vi "Robot Global Data.vi"() -> ()   [LabVIEW 2018]
doc: "This global VI can contain as many global variables as you need. Place a control on the panel, give it a good name. To read or write to it from a VI, drag the icon to the diagram of that VI. You can also drag from the project. Click on the node to change which global you access. You shouldn't have multiple locations writing to a global or it will cause a race-condition."
uses:
  <vilib>/Rock Robotics/WPI/Camera/WPI_CameraImageSize.ctl
  <vilib>/Rock Robotics/WPI/DriverStation/WPI_DriverStationRobotMode2.ctl
  Infrastructure/Joystick Controls.ctl
  Drivebase/Drive Motion Magic Setpoints.ctl
  <vilib>/Rock Robotics/WPI/ThirdParty/Phoenix-LabVIEW/Motor Controller/Controls/CTRE_Phoenix_MotorControl_ControlMode.ctl
panel:
  out "4bar setpoint/immediate value":T2 {"Control Mode" items=["PercentOutput"=0, "Position"=1, "Velocity"=2, "Current"=3, "Follower"=5, "MotionProfile"=6, "MotionMagic"=7, "MotionProfileArc"=10, "Disabled"=15]}
  in  "Drive Motor Values":T3
  in  "Manual Has Overridden Auton":bool
  in  "Drive MM Setpoints":T4
  in  "Step Auton Drive has Completed":i32
  in  "Joystick Controls":T5={"Driver Left Joystick X"=0.0, "Driver Left Joystick Y"=0.0, "Driver A Button"=FALSE, "Driver B Button"=FALSE, "Driver X Button"=FALSE, "Driver Y Button"=FALSE, "Driver Left Bumper"=FALSE, "Driver Right Bumper"=FALSE, "Driver View Button"=FALSE, "Driver Menu Button"=FALSE, "Driver Left Joystick Press"=FALSE, "Driver Right Joystick Press"=FALSE, "Driver Left Trigger"=0.0, "Driver Right Joystick X"=0.0, "Driver Right Joystick Y"=0.0, "Driver Right Trigger"=0.0, "Operator Left Joystick X"=0.0, "Operator Left Joystick Y"=0.0, "Operator A Button"=FALSE, "Operator B Button"=FALSE, "Operator X Button"=FALSE, "Operator Y Button"=FALSE, "Operator Left Bumper"=FALSE, "Operator Right Bumper"=FALSE, "Operator View Button"=FALSE, "Operator Menu Button"=FALSE, "Operator Left Joystick Press"=FALSE, "Operator Right Joystick Press"=FALSE, "Operator Left Trigger"=0.0, "Operator Right Joystick X"=0.0, "Operator Right Joystick Y"=0.0, "Operator Right Trigger"=0.0, "Driver D-Pad"=-1, "Operator D-Pad"=-1}
  in  "Robot Mode":T6
  in  "image size":T7=enum."320x240"
  in  "Enable Vision":bool
  # "AUTON"
  # "Typedef\nWriten to in Autonomous independant"
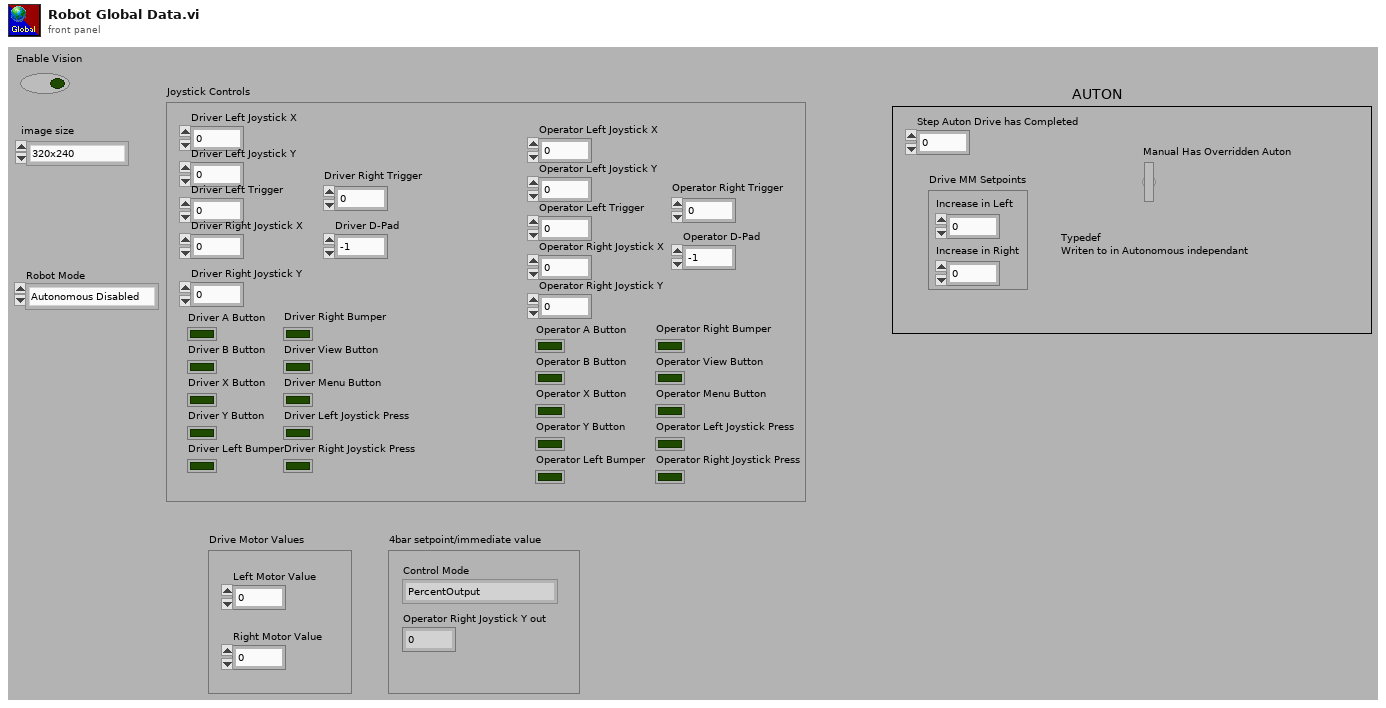
[diagram p1: front panel]
types:
  T1 = typedef "CTRE_Phoenix_MotorControl_ControlMode.ctl" = u16
  T2 = cluster{"Control Mode":T1, "Operator Right Joystick Y out":dbl}
  T3 = cluster{"Left Motor Value":dbl, "Right Motor Value":dbl}
  T4 = typedef "Drive Motion Magic Setpoints.ctl" = cluster{"Increase in Left":dbl, "Increase in Right":dbl}
  T5 = typedef "Joystick Controls.ctl" = cluster{"Driver Left Joystick X":dbl, "Driver Left Joystick Y":dbl, "Driver A Button":bool, "Driver B Button":bool, "Driver X Button":bool, "Driver Y Button":bool, "Driver Left Bumper":bool, "Driver Right Bumper":bool, "Driver View Button":bool, "Driver Menu Button":bool, "Driver Left Joystick Press":bool, "Driver Right Joystick Press":bool, "Driver Left Trigger":dbl, "Driver Right Joystick X":dbl, "Driver Right Joystick Y":dbl, "Driver Right Trigger":dbl, "Operator Left Joystick X":dbl, "Operator Left Joystick Y":dbl, "Operator A Button":bool, "Operator B Button":bool, "Operator X Button":bool, "Operator Y Button":bool, "Operator Left Bumper":bool, "Operator Right Bumper":bool, "Operator View Button":bool, "Operator Menu Button":bool, "Operator Left Joystick Press":bool, "Operator Right Joystick Press":bool, "Operator Left Trigger":dbl, "Operator Right Joystick X":dbl, "Operator Right Joystick Y":dbl, "Operator Right Trigger":dbl, "Driver D-Pad":i16, "Operator D-Pad":i16}
  T6 = typedef "WPI_DriverStationRobotMode2.ctl" = enum16{"Autonomous Disabled", "Autonomous Enabled", "Teleop Disabled", "Teleop Enabled", "Disconnected", "Finish", "Test Disabled", "Test Enabled", "Emergency Stopped"}
  T7 = typedef "WPI_CameraImageSize.ctl" = enum16{"640x480", "320x240", "160x120", "Custom"}
diagram:
